vi "分隔栏.vi"   [LabVIEW 2010]
doc: "本VI是为《我和LabVIEW》一书编写的示例。\n关于本书的介绍请参考网页：\nhttp://ruanqizhen.spaces.live.com/blog/cns!5852D4F797C53FB6!4310.entry"
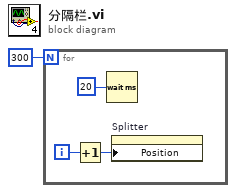
[diagram p0: block diagram]
diagram:
  n1 = for {
    N: 300 -> [_]
    i -> [w3]
    n2 = Increment(x=w3) -> (x+1=w2:i32)
    n3 = Wait (ms)(milliseconds to wait=u32 20) -> ()  [unwired: 1 out]
    n4 = property on="Splitter" class="Splitter"("Position"=w2) -> ()  [unwired: 2 in, 2 out]
  }
